vi "Calibration Directives.vi"() -> (0 "Input Channels":string, 1 "Output Channels":string, 2 "Output Waveforms":waveform(dbl)[](array[waveform]))   [LabVIEW 2013]
uses:
  <vilib>/Waveform/WDTOps.llb/WDT Append Waveforms DBL.vi
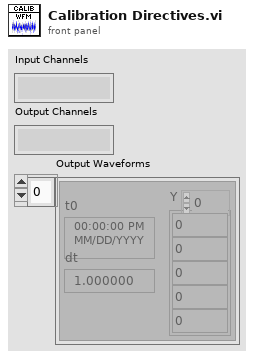
[diagram p1: front panel]
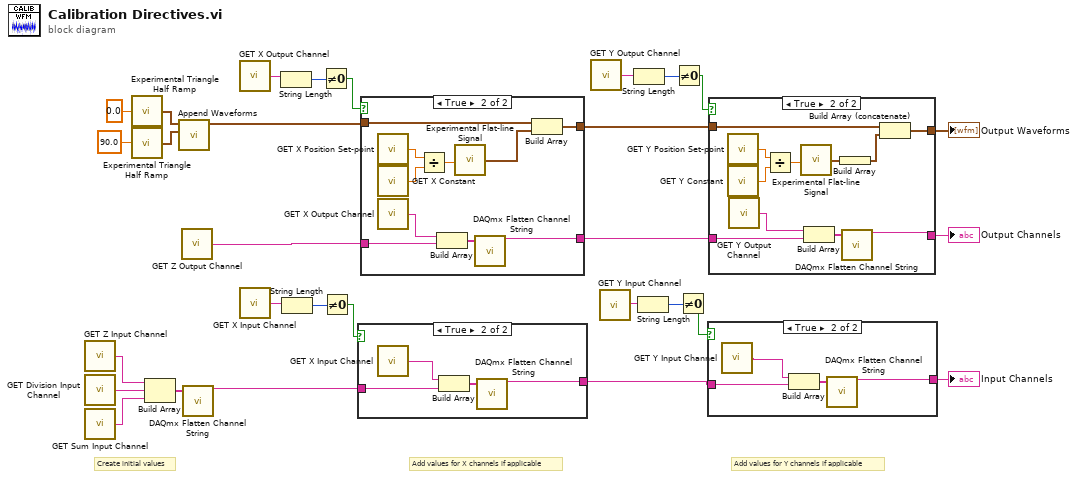
[diagram p0: block diagram]
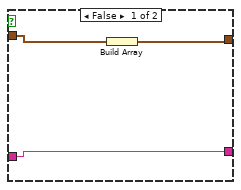
[diagram p5: hidden frame]
diagram:
  # "Add values for Y channels if applicable"
  # "Add values for X channels if applicable"
  # "Create initial values"
  n1 = call "GET Z Input Channel.vi"() -> ("Z Input Channel"=w13:string)
  n2 = call "GET Division Input Channel.vi"() -> ("Division Input Channel"=w12:string)
  n3 = call "GET Sum Input Channel.vi"() -> ("Sum Input Channel"=w11:string)
  n4 = call "Experimental Triangle Half Ramp.vi"("Phase Offset"=0.0) -> ("Half Triangle"=w4:waveform(dbl))
  n5 = call "Experimental Triangle Half Ramp.vi"("Phase Offset"=90.0) -> ("Half Triangle"=w1:waveform(dbl))
  n6 = Build Array(w13, w12, w11) -> (w14:string[])
  n7 = call-poly <vilib>:"Append Waveforms.vi"("waveform B"=w1, "waveform A"=w4) -> ("waveform out"=w26:waveform(dbl))  [unwired: 8 in, 1 out]
  n8 = call "GET Z Output Channel.vi"() -> ("Z Output Channel"=w21:string)
  n9 = call <vilib>:"DAQmx Flatten Channel String.vi"("names in"=w14) -> ("names out"=w10:string)  [unwired: 13 in, 1 out]
  n10 = call "GET X Output Channel.vi"() -> ("X Output Channel"=w29:string)
  n11 = call "GET X Input Channel.vi"() -> ("X Input Channel"=w17:string)
  n12 = String Length(string=w29) -> (length=w28:i32)
  n13 = String Length(string=w17) -> (length=w19:i32)
  n14 = Not Equal To 0?(x=w28) -> (x != 0?=w27:bool)
  n15 = Not Equal To 0?(x=w19) -> (x != 0?=w15:bool)
  n16 = case shown="True" w15 {
    tunnel: w10 -> [w30 w33]
    tunnel: [w30 w31] -> w8
    frame False {
    }
    frame True {
      n17 = call "GET X Input Channel.vi"() -> ("X Input Channel"=w32:string)
      n18 = Build Array(w32, w33) -> (w34:string[])
      n19 = call <vilib>:"DAQmx Flatten Channel String.vi"("names in"=w34) -> ("names out"=w31:string)  [unwired: 13 in, 1 out]
    }
  }
  n20 = case shown="True" w27 {
    tunnel: w26 -> [w37 w44]
    tunnel: [w36 w43] -> w22
    tunnel: w21 -> [w35 w40]
    tunnel: [w35 w39] -> w20
    frame False {
      n21 = Build Array(w37) -> (w36:waveform(dbl)[])
    }
    frame True {
      n22 = call "GET X Position Set-point.vi"() -> ("X Position Set-point"=w45:dbl)
      n23 = call "GET X Constant.vi"() -> ("X Constant"=w46:dbl)
      n24 = call "GET X Output Channel.vi"() -> ("X Output Channel"=w42:string)
      n25 = Divide(x=w45, y=w46) -> (x/y=w47:dbl)
      n26 = Build Array(w42, w40) -> (w41:string[])
      n27 = call "Experimental Flat-line Signal.vi"("Flatline Offset"=w47) -> ("Flatline Signal"=w38:waveform(dbl))
      n28 = call <vilib>:"DAQmx Flatten Channel String.vi"("names in"=w41) -> ("names out"=w39:string)  [unwired: 13 in, 1 out]
      n29 = Build Array(w44, w38) -> (w43:waveform(dbl)[])
    }
  }
  n30 = call "GET Y Output Channel.vi"() -> ("Y Output Channel"=w24:string)
  n31 = call "GET Y Input Channel.vi"() -> ("Y Input Channel"=w16:string)
  n32 = String Length(string=w24) -> (length=w25:i32)
  n33 = String Length(string=w16) -> (length=w18:i32)
  n34 = Not Equal To 0?(x=w25) -> (x != 0?=w23:bool)
  n35 = Not Equal To 0?(x=w18) -> (x != 0?=w9:bool)
  n36 = case shown="True" w9 {
    tunnel: w8 -> [w48 w51]
    tunnel: [w48 w50] -> w5
    frame False {
    }
    frame True {
      n37 = call "GET Y Input Channel.vi"() -> ("Y Input Channel"=w49:string)
      n38 = Build Array(w49, w51) -> (w52:string[])
      n39 = call <vilib>:"DAQmx Flatten Channel String.vi"("names in"=w52) -> ("names out"=w50:string)  [unwired: 13 in, 1 out]
    }
  }
  "Input Channels" <- w5
  n40 = case shown="True" w23 {
    tunnel: w22 -> [w54 w60]
    tunnel: [w54 w59] -> w7
    tunnel: w20 -> [w53 w56]
    tunnel: [w53 w55] -> w6
    frame False {
    }
    frame True {
      n41 = call "GET Y Position Set-point.vi"() -> ("Y Position Set-point"=w64:dbl)
      n42 = call "GET Y Constant.vi"() -> ("Y Constant"=w63:dbl)
      n43 = call "GET Y Output Channel.vi"() -> ("Y Output Channel"=w57:string)
      n44 = Divide(x=w64, y=w63) -> (x/y=w65:dbl)
      n45 = call "Experimental Flat-line Signal.vi"("Flatline Offset"=w65) -> ("Flatline Signal"=w62:waveform(dbl))
      n46 = Build Array(w57, w56) -> (w58:string[])
      n47 = Build Array(w62) -> (w61:waveform(dbl)[])
      n48 = call <vilib>:"DAQmx Flatten Channel String.vi"("names in"=w58) -> ("names out"=w55:string)  [unwired: 13 in, 1 out]
      n49 = Build Array (concatenate)(w60, w61) -> (w59:waveform(dbl)[])
    }
  }
  "Output Channels" <- w6
  "Output Waveforms" <- w7
